vi "Cleanup.vi"(8 "error in (no error)":errorcluster, 11 "Class In":refnum<class "Recipe Editor.lvclass">) -> (0 "error out":errorcluster)   [LabVIEW 2018, in "Temp Recipe.lvlib" / "Recipe Editor.lvclass"]
uses:
  Recipe Editor.lvclass
  Recipe Editor.lvclass/Recipe Editor.ctl
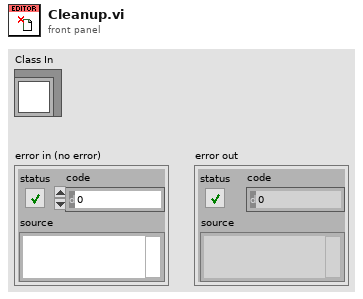
[diagram p1: front panel]
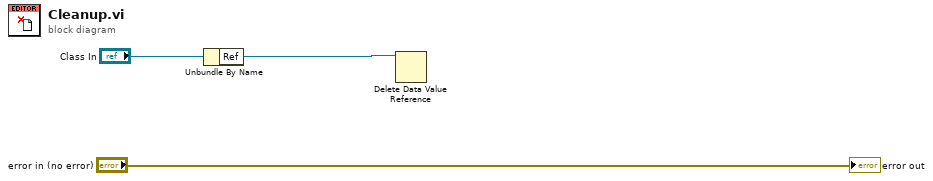
[diagram p0: block diagram]
diagram:
  n1 = Unbundle By Name("Class In") -> ("Ref"=w1:refnum<data-value>)
  n2 = Delete Data Value Reference(data value reference=w1) -> ()  [unwired: 1 in, 2 out]
  "error out" <- "error in (no error)"
